vi "GetPowerReading.vi"(8 "error in (no error)":errorcluster, 11 "Laser Diode Controller in":refnum<class "KLD101.lvclass">) -> (0 "error out":errorcluster, 2 "powerReading":dbl, 3 "Laser Diode Controller out":refnum<class "KLD101.lvclass">)   [LabVIEW 2016, in "Laser Diode Controller.lvlib" / "KLD101.lvclass"]
uses:
  KLD101.lvclass
  KLD101.lvclass/KLD101.ctl
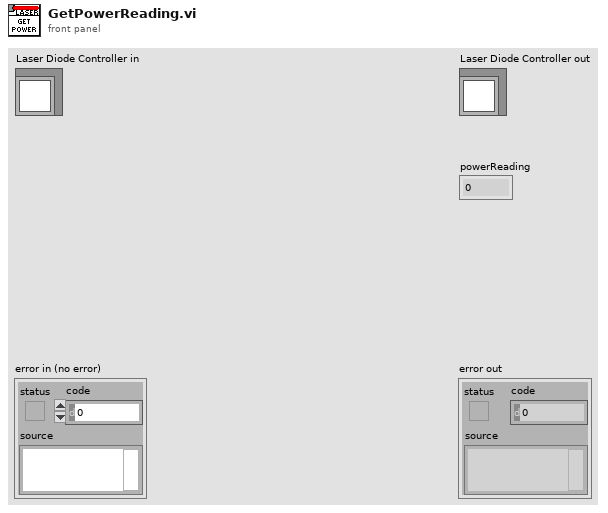
[diagram p1: front panel]
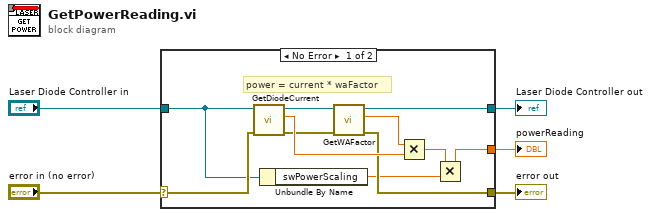
[diagram p0: block diagram]
diagram:
  n1 = case shown="No Error" "error in (no error)" {
    selector: "error in (no error)" -> [w11 w18]
    tunnel: [w10 w18] -> w4
    tunnel: [w15 w17] -> w2
    tunnel: "Laser Diode Controller in" -> [w7 w17]
    tunnel: [w8 _] -> w1
    frame No Error {
      # "power = current * waFactor"
      n2 = call-dynamic "GetDiodeCurrent.vi"("error in (no error)"=w11, "Laser Diode Controller in"=w7) -> ("error out"=w12:errorcluster, "diodeCurrent"=w13:dbl, "Laser Diode Controller out"=w16:refnum<class "KLD101.lvclass">)  [unwired: 7 in]
      n3 = Unbundle By Name(w7) -> ("swPowerScaling"=w6:dbl)
      n4 = call-dynamic "GetWAFactor.vi"("error in (no error)"=w12, "Laser Diode Controller in"=w16) -> ("error out"=w10:errorcluster, "waFactor"=w14:dbl, "Laser Diode Controller out"=w15:refnum<class "KLD101.lvclass">)  [unwired: 7 in]
      n5 = Multiply(x=w14, y=w13) -> (x*y=w9:dbl)
      n6 = Multiply(x=w9, y=w6) -> (x*y=w8:dbl)
    }
    frame Error {
    }
  }
  "error out" <- w4
  "Laser Diode Controller out" <- w2
  "powerReading" <- w1
